vi "CS-4 Reset.vi"(8 "error in (no error)":errorcluster, 11 "VISA session":refnum<visa-resource-name>) -> (0 "error out":errorcluster, 3 "dup VISA session":refnum<visa-resource-name>)   [LabVIEW 2020]
doc: "This VI resets the instrument, and then sends a set of default setup commands to the instrument. If a Reset command is not supported, it will return a warning."
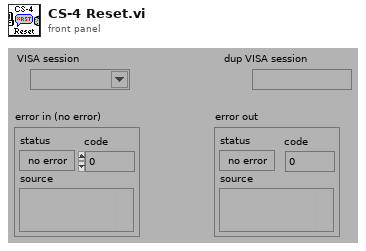
[diagram p1: front panel]
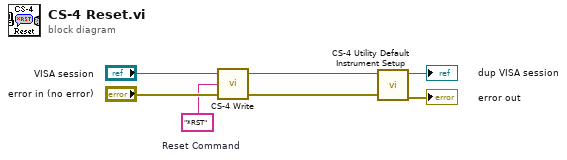
[diagram p0: block diagram]
diagram:
  w3 = "*RST"  # Reset Command
  n1 = call "CS-4 Write.vi"("error in (no error)"="error in (no error)", "write buffer (\"\")"=w3, "VISA session"="VISA session") -> ("error out"=w1:errorcluster, "dup VISA session"=w2:refnum<visa-resource-name>)  [unwired: 1 out]
  n2 = call "CS-4 Utility Default Instrument Setup.vi"("error in (no error)"=w1, "VISA session"=w2) -> ("error out"=→"error out":errorcluster, "dup VISA session"=→"dup VISA session":refnum<visa-resource-name>)  [unwired: 8 in]
